vi "PowerOff.vi"(0 "Universal Robot.lvclass in":refnum<class "Universal Robot.lvclass">, 5 "error in (no error)":errorcluster) -> (14 "Universal Robot.lvclass out":refnum<class "Universal Robot.lvclass">, 19 "error out":errorcluster)   [LabVIEW 2016, in "Universal Robot.lvclass"]
uses:
  Universal Robot.lvclass
  Universal Robot.lvclass/Universal Robot.ctl
  RobotMode.ctl
  DashboardServer/Dashboard Server.lvclass
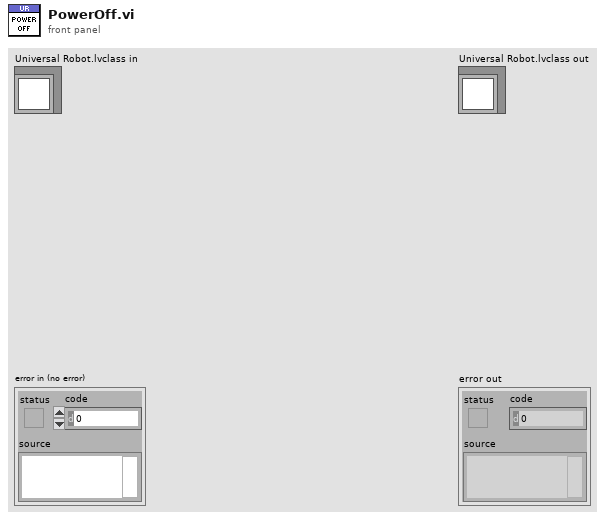
[diagram p1: front panel]
types:
  T1 = typedef "Universal Robot.lvclass/RobotMode.ctl" = enum16{"INVALID", "NO_CONTROLLER", "DISCONNECTED", "CONFIRM_SAFETY", "BOOTING", "POWER_OFF", "POWER_ON", "IDLE", "BACKDRIVE", "RUNNING"}
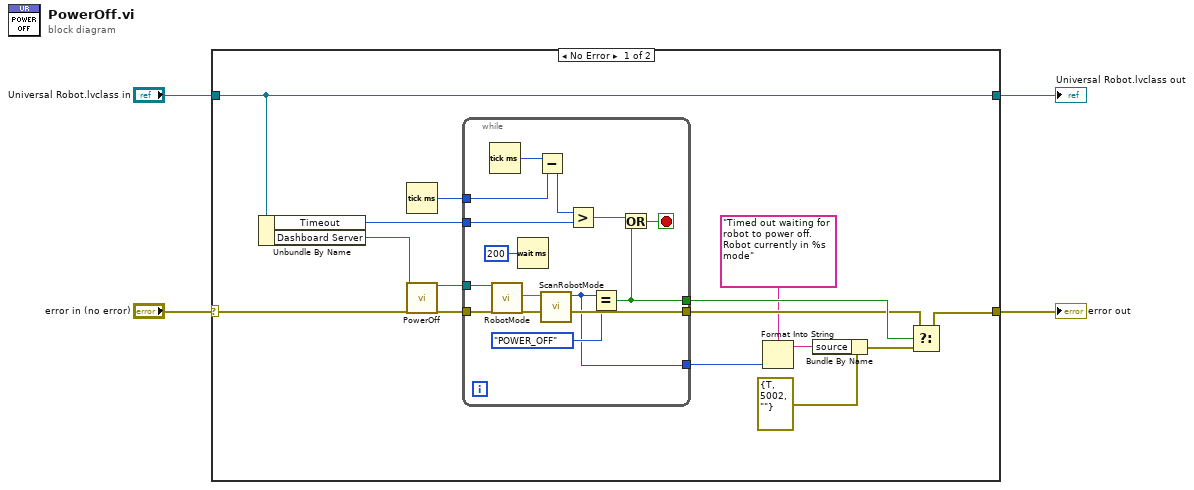
[diagram p0: block diagram]
diagram:
  n1 = case shown="No Error" "error in (no error)" {
    selector: "error in (no error)" -> [w8 w35]
    tunnel: [w19 w35] -> w3
    tunnel: "Universal Robot.lvclass in" -> [w17 w34]
    tunnel: [w17 w34] -> w1
    frame No Error {
      n2 = Unbundle By Name(w17) -> ("Timeout"=w18:u32, "Dashboard Server"=w5:refnum<class "Dashboard Server.lvclass">)
      n3 = Tick Count (ms)() -> (millisecond timer value=w16:u32)
      n4 = call-dynamic "PowerOff.vi"("DashboardServer in"=w5, "error in (no error)"=w8) -> ("DashboardServer out"=w6:refnum<class "Dashboard Server.lvclass">, "error out"=w7:errorcluster)  [unwired: 16 in]
      n5 = while {
        tunnel: w6 -> [w32]
        tunnel: w7 -> [w33]
        tunnel: [w31] -> w14
        tunnel: w18 -> [w29]
        tunnel: w16 -> [w28]
        tunnel: [w23] -> w15
        tunnel: [w20] -> w13
        stop <- w24 stop-if-true
        n6 = Tick Count (ms)() -> (millisecond timer value=w27:u32)
        n7 = call-dynamic "RobotMode.vi"("DashboardServer in"=w32, "error in (no error)"=w33) -> ("robotMode"=w22:string, "error out"=w31:errorcluster)  [unwired: 15 in, 1 out]
        n8 = Wait (ms)(milliseconds to wait=u32 200) -> ()  [unwired: 1 out]
        n9 = Subtract(x=w27, y=w28) -> (x-y=w26:u32)
        n10 = call "ScanRobotMode.vi"("robotMode in"=w22) -> ("robotMode out"=w20:T1)  [unwired: 10 in]
        n11 = Greater?(x=w26, y=w29) -> (0:w25:bool)
        n12 = Equal?(x=w20, y=RobotMode."POWER_OFF") -> (x = y?=w23:bool)
        n13 = Or(x=w25, y=w23) -> (x .or. y?=w24:bool)
      }
      n14 = Format Into String(format string="Timed out waiting for robot to power off. Robot currently in %s mode", w13) -> (resulting string=w11:string)  [unwired: 2 in, 1 out]
      n15 = Bundle By Name(cluster=errorcluster {"status"=TRUE, "code"=5002, "source"=""} ("error constant"), "source"=w11) -> (w10:errorcluster)
      n16 = Select(t=w14, s=w15, f=w10) -> (s? t:f=w19:errorcluster)
    }
    frame Error {
    }
  }
  "error out" <- w3
  "Universal Robot.lvclass out" <- w1
